vi "Validate Instrument Revision.vi"(0 "VISA resource name":refnum<visa-resource-name>, 11 "error in (no error)":errorcluster) -> (4 "VISA resource name out":refnum<visa-resource-name>, 6 "Firmware Version":string, 10 "Model Number":enum16{"310XAC", "320XAC", "340XAC", "360XAC"}(ring), 15 "error out":errorcluster)   [LabVIEW 2016, in "APT 300XAC Series.lvlib"]
doc: "Queries the instrument for the model number and firmware revision and validates them."
uses:
  APT 300XAC Series.lvlib
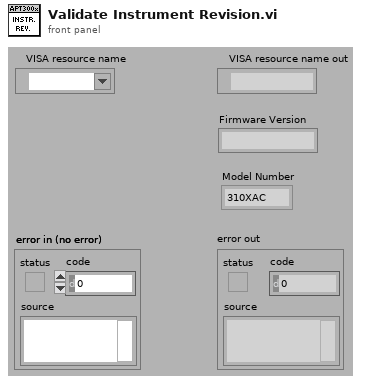
[diagram p1: front panel]
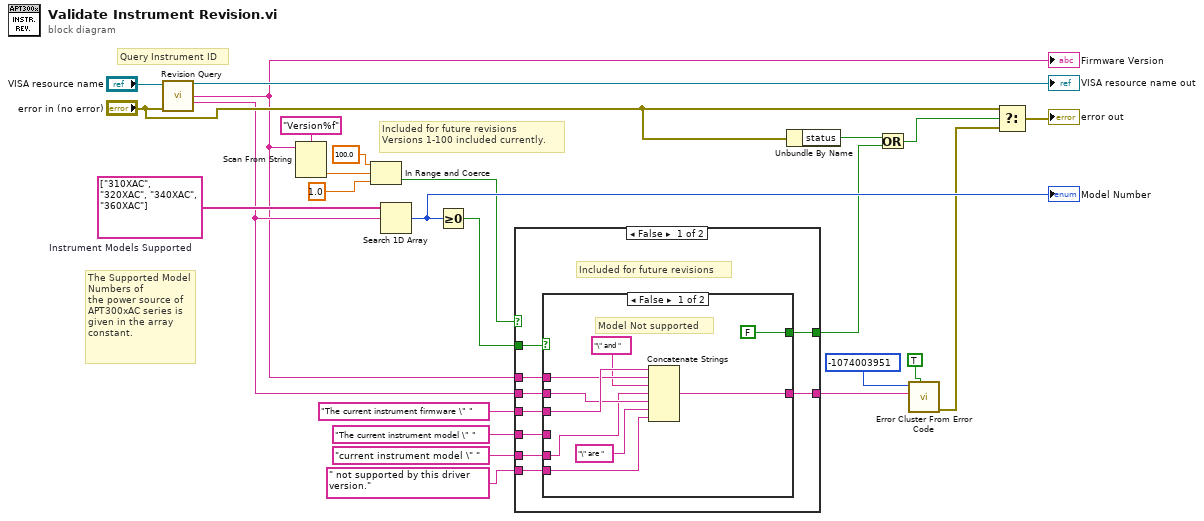
[diagram p0: block diagram]
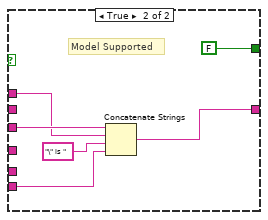
[diagram p2: hidden frame]
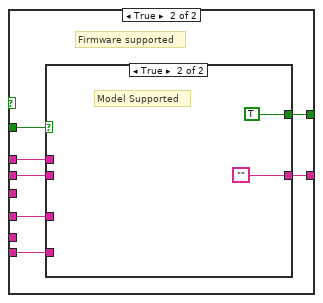
[diagram p3: hidden frame]
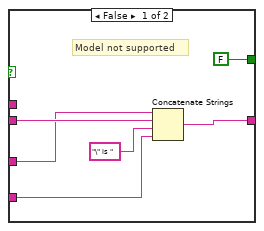
[diagram p4: hidden frame]
diagram:
  w24 = string[] ["310XAC", "320XAC", "340XAC", "360XAC"]  # Instrument Models Supported
  # "Included for future revisions\nVersions 1-100 included currently."
  # "The Supported Model Numbers of\nthe power source of APT300xAC series is given in the array constant."
  # "Query Instrument ID"
  n1 = call "Revision Query.vi"("VISA resource name"="VISA resource name", "error in (no error)"="error in (no error)") -> ("VISA resource name out"=→"VISA resource name out":refnum<visa-resource-name>, "Instrument Firmware Revision"=w1:string, "Instrument Model"=w4:string)  [unwired: 9 in, 2 out]
  "Firmware Version" <- w1
  n2 = Scan From String(format string="Version%f", input string=w1) -> (output 1=w3:dbl)  [unwired: 3 in, 3 out]
  n3 = In Range and Coerce(upper limit=100.0 ("y"), x=w3, lower limit=1.0 ("y")) -> (In Range?=w7:bool)  [unwired: 1 out]
  n4 = Search 1D Array(1D array=w24, element=w4) -> (index of element=w25:i32)  [unwired: 1 in]
  "Model Number" <- w25
  n5 = Greater Or Equal To 0?(x=w25) -> (x >= 0?=w17:bool)
  n6 = case shown="False" w7 {
    tunnel: w17 -> [w33 w56]
    tunnel: w4 -> [w34 w55]
    tunnel: w1 -> [w32 w54]
    tunnel: " not supported by this driver version." ("Source (VI Name)") -> [w31 w52]
    tunnel: "The current instrument model \" " ("Source (VI Name)") -> [w30 w53]
    tunnel: "The current instrument firmware \" " ("Source (VI Name)") -> [w29 _]
    tunnel: [w28 w51] -> w13
    tunnel: [w27 w50] -> w11
    tunnel: "current instrument model \" " ("Source (VI Name)") -> [w26 _]
    frame False {
      # "Included for future revisions"
      n7 = case shown="False" w33 {
        tunnel: w34 -> [w41 _]
        tunnel: w32 -> [w42 w48]
        tunnel: w31 -> [w40 w46]
        tunnel: w30 -> [_ _]
        tunnel: w29 -> [w43 w49]
        tunnel: [w37 w44] -> w28
        tunnel: [FALSE ("show call chain? (False)") FALSE ("show call chain? (False)")] -> w27
        tunnel: w26 -> [w35 _]
        frame False {
          # "Model Not supported"
          n8 = Concatenate Strings(w43, w42, "\" and " ("string"), w35, w41, "\" are " ("Source (VI Name)"), w40) -> (w37:string)
        }
        frame True {
          # "Model Supported"
          n9 = Concatenate Strings(w49, w48, "\" is " ("string"), w46) -> (w44:string)
        }
      }
    }
    frame True {
      # "Firmware supported"
      n10 = case shown="True" w56 {
        tunnel: w55 -> [w61 _]
        tunnel: w54 -> [_ _]
        tunnel: w53 -> [w60 _]
        tunnel: w52 -> [w59 _]
        tunnel: [w58 ""] -> w51
        tunnel: [FALSE TRUE] -> w50
        frame False {
          # "Model not supported"
          n11 = Concatenate Strings(w60, w61, "\" is " ("string"), w59) -> (w58:string)
        }
        frame True {
          # "Model Supported"
        }
      }
    }
  }
  n12 = Unbundle By Name("error in (no error)") -> ("status"=w10:bool)
  n13 = Or(x=w10, y=w11) -> (x .or. y?=w9:bool)
  n14 = call <vilib>:"Error Cluster From Error Code.vi"("show call chain? (False)"=TRUE, "error message (\"\")"=w13, "error code (0)"=-1074003951 ("Code")) -> ("error out"=w21:errorcluster)  [unwired: 6 in]
  n15 = Select(t="error in (no error)", s=w9, f=w21) -> (s? t:f=→"error out":errorcluster)
